vi "DSC.vi"() -> ()   [LabVIEW 2017]
uses:
  Program Files (x86)/National Instruments/LabVIEW 2017/examples/lvdsc/XControls/Animator/Control/AnimatorXControl.xctl
panel:
  in  "AnimatorXControl":u32(xcontrol)
  in  "Boolean 13":bool
  out "Boolean 12":bool
  out "Boolean 11":bool
  out "Boolean 5":bool
  out "Tank":dbl(slide) scale=0.0..10.0
  in  "stop":bool
  in  "Boolean 10":bool
  out "Boolean 9":bool
  out "Boolean 8":bool
  out "Boolean 7":bool
  out "Boolean 6":bool
  out "Boolean 4":bool
  out "Boolean 3":bool
  out "Boolean 2":bool
  out "Boolean":bool
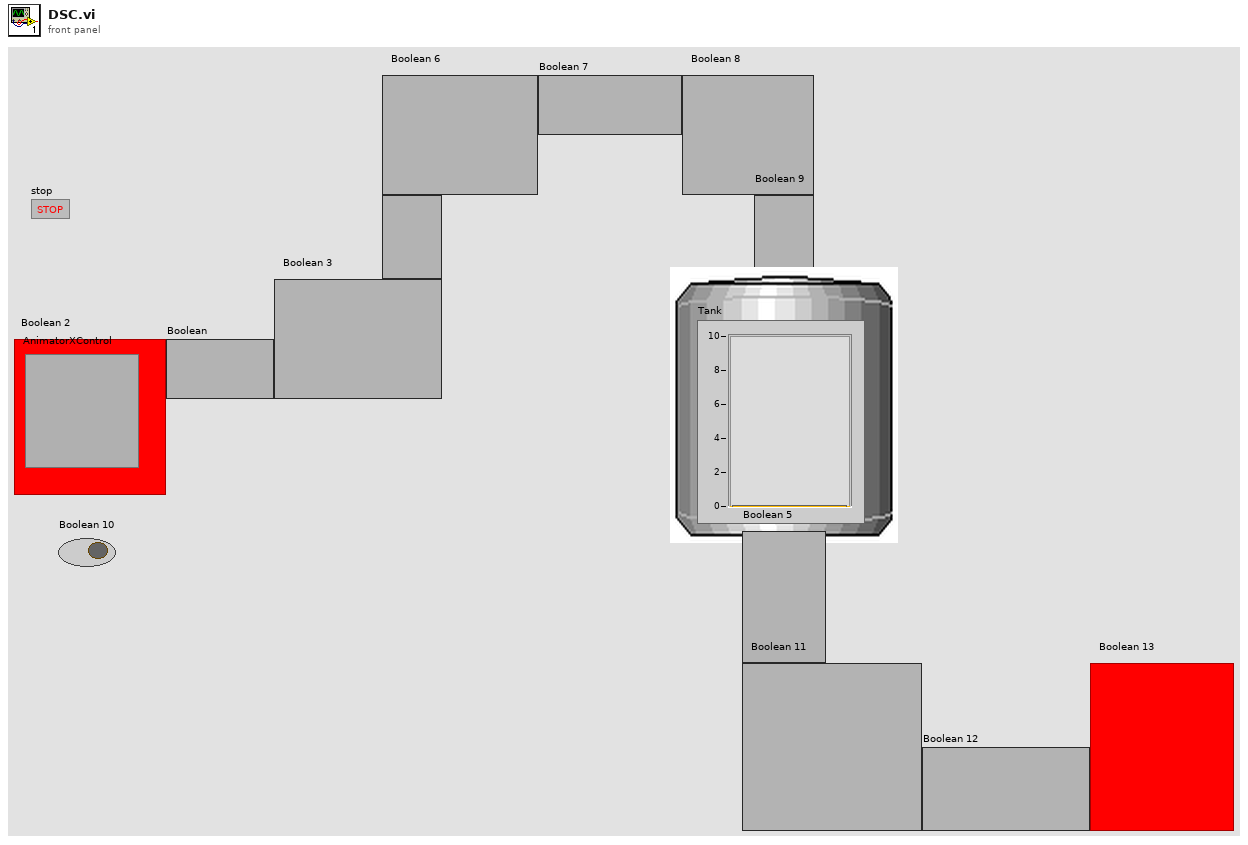
[diagram p1: front panel]
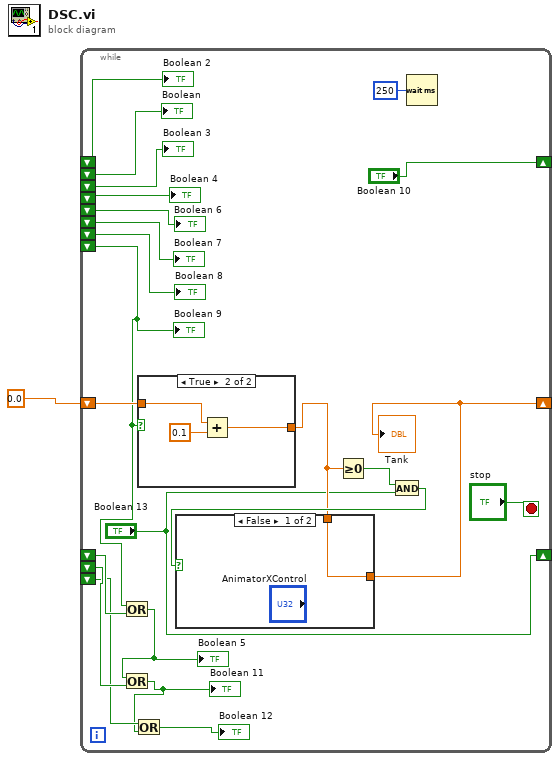
[diagram p0: block diagram]
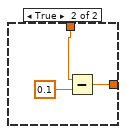
[diagram p2: hidden frame]
diagram:
  n1 = while {
    shift-right: ["Boolean 10"] -> _
    shift-left: _ -> [w22]
    shift-left: _ -> [w20]
    shift-left: _ -> [w21]
    shift-left: _ -> [w19]
    shift-left: _ -> [w18]
    shift-left: _ -> [w17]
    shift-left: _ -> [w16]
    shift-left: _ -> [w8]
    shift-right: [w10] -> _
    shift-left: 0.0 -> [w14]
    shift-right: ["Boolean 13"] -> _
    shift-left: _ -> [w7]
    shift-left: _ -> [w5]
    shift-left: _ -> [w3]
    stop <- "stop" stop-if-true
    n2 = Or(x=w8, y=w7) -> (x .or. y?=w6:bool)
    "Boolean 5" <- w6
    n3 = Or(x=w6, y=w5) -> (x .or. y?=w2:bool)
    "Boolean 11" <- w2
    n4 = Or(x=w3, y=w2) -> (x .or. y?=→"Boolean 12":bool)
    n5 = case shown="True" w8 {
      tunnel: w14 -> [w29 w32]
      tunnel: [w29 w30] -> w11
      frame False {
      }
      frame True {
        n6 = Add(x=w32, y=0.1) -> (x+y=w30:dbl)
      }
    }
    n7 = Greater Or Equal To 0?(x=w11) -> (x >= 0?=w13:bool)
    n8 = And(x=w13, y="Boolean 13") -> (x .and. y?=w12:bool)
    n9 = case shown="False" w12 {
      tunnel: w11 -> [w25 w28]
      tunnel: [w25 w26] -> w10
      frame False {
      }
      frame True {
        n10 = Subtract(x=w28, y=0.1) -> (x-y=w26:dbl)
      }
    }
    "Tank" <- w10
    n11 = Wait (ms)(milliseconds to wait=u32 250) -> ()  [unwired: 1 out]
    "Boolean" <- w21
    "Boolean 2" <- w22
    "Boolean 3" <- w20
    "Boolean 4" <- w19
    "Boolean 6" <- w18
    "Boolean 7" <- w17
    "Boolean 8" <- w16
    "Boolean 9" <- w8
  }
